vi "Get Case Struct Terminals.vi"(8 "Error In":errorcluster, 11 "Case Structure in":refnum<vi>) -> (0 "Error Out":errorcluster, 2 "Tunnels[]":refnum<vi>[](array[refnum]), 3 "Case Structure out":refnum<vi>)   [LabVIEW 2019, in "gRPC Scripting Tools.lvlib"]
doc: "Use this template to build a VI to use as a subVI."
uses:
  gRPC Scripting Tools.lvlib
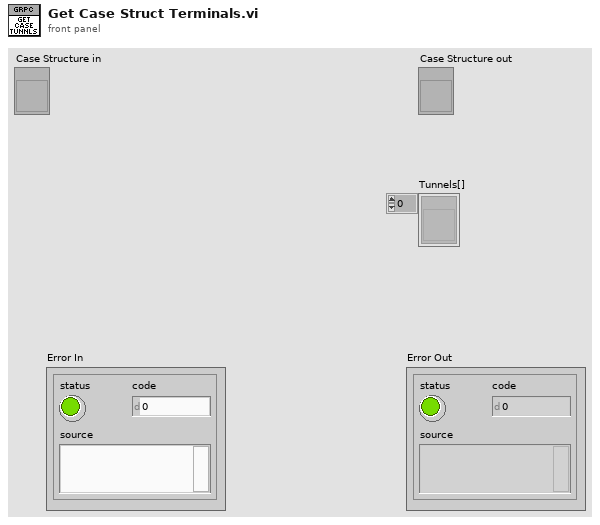
[diagram p1: front panel]
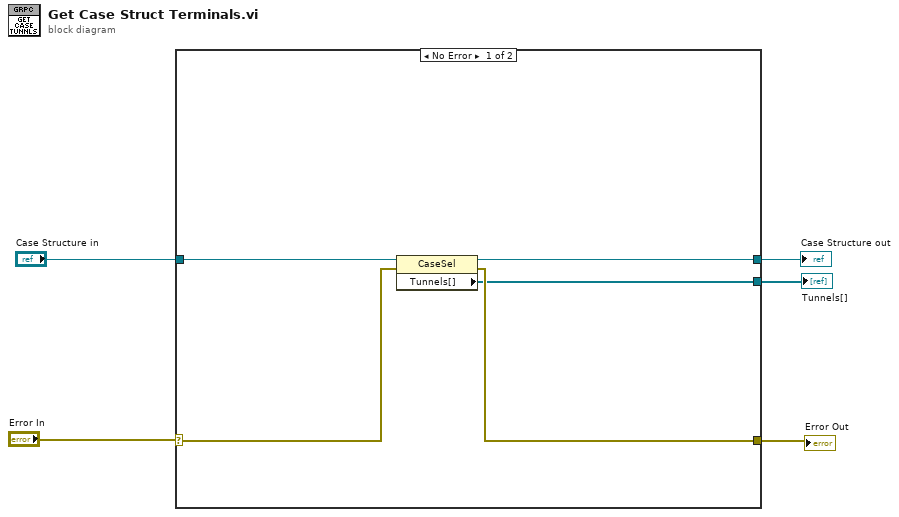
[diagram p0: block diagram]
diagram:
  n1 = case shown="No Error" "Error In" {
    selector: "Error In" -> [w10 w12]
    tunnel: [w9 w12] -> w4
    tunnel: "Case Structure in" -> [w8 w11]
    tunnel: [w7 w11] -> w2
    tunnel: [w6 _] -> w1
    frame No Error {
      n2 = property class="CaseSel"(reference=w8, error in=w10) -> (reference out=w7:refnum<vi>, error out=w9:errorcluster, "Tunnels[]"=w6:refnum<vi>[])
    }
    frame Error {
    }
  }
  "Error Out" <- w4
  "Case Structure out" <- w2
  "Tunnels[]" <- w1
